vi "Script Flat to Rich Message Conversion.vi"(8 "error in (no error)":errorcluster, 9 "message metadata":T1, 10 "vi in":refnum<vi>, 11 "library in":refnum<vi>) -> (0 "error out":errorcluster, 2 "vi out":refnum<vi>, 3 "library out":refnum<vi>)   [LabVIEW 2019, in "gRPC Template Creation Utility.lvlib"]
uses:
  gRPC Template Creation Utility.lvlib
  TypeDefs/Message Metadata (Scripting).ctl
  TypeDefs/Message Element Metadata (Scripting).ctl
  TypeDefs/Message Element Type.ctl
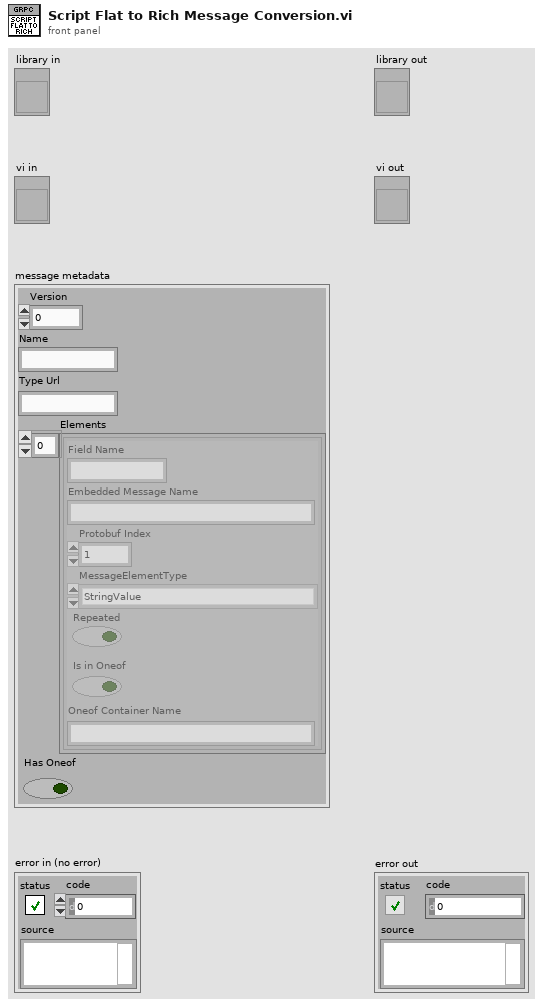
[diagram p1: front panel]
types:
  T1 = typedef "gRPC Template Creation Utility.lvlib/Message Metadata (Scripting).ctl" = cluster{"Version":i32, "Name":string, "Type Url":string, "Elements":T2[], "Has Oneof":bool}
  T2 = typedef "gRPC Template Creation Utility.lvlib/Message Element Metadata (Scripting).ctl" = cluster{"Field Name":string, "Embedded Message Name":string, "Protobuf Index":i32, "MessageElementType":T3, "Repeated":bool, "Is in Oneof":bool, "Oneof Container Name":string}
  T3 = typedef "gRPC Template Creation Utility.lvlib/Message Element Type.ctl" = enum32{"Int32Value", "FloatValue", "DoubleValue", "BoolValue", "StringValue", "MessageValue", "Int64Value", "UInt32Value", "UInt64Value", "EnumValue", "Bytes", "Fixed64", "Fixed32", "SFixed64", "SFixed32", "SInt64", "SInt32"}
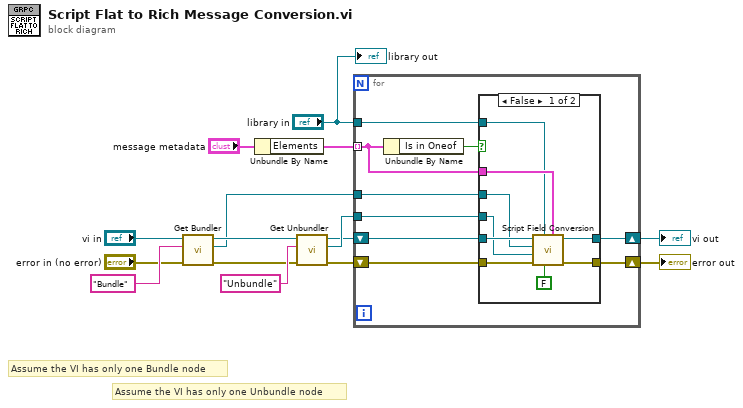
[diagram p0: block diagram]
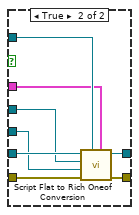
[diagram p2: hidden frame]
diagram:
  # "Assume the VI has only one Bundle node"
  # "Assume the VI has only one Unbundle node"
  n1 = call "Get Bundler.vi"("error in (no error)"="error in (no error)", "label"="Bundle" ("Class Name"), "owner vi in"="vi in") -> ("error out"=w7:errorcluster, "bundler ref"=w5:refnum<vi>, "owner vi out"=w8:refnum<vi>)  [unwired: 5 in, 1 out]
  n2 = Unbundle By Name("message metadata") -> ("Elements"=w3:T2[])
  n3 = call "Get Unbundler.vi"("error in (no error)"=w7, "Label"="Unbundle" ("Class Name"), "Owner VI in"=w8) -> ("error out"=w4:errorcluster, "Unbundler Refnum"=w10:refnum<vi>, "Owner VI out"=w9:refnum<vi>)  [unwired: 5 in, 1 out]
  n4 = for {
    tunnel: w3 -> [w16] mode=indexing
    tunnel: w5 -> [w24]
    tunnel: w10 -> [w23]
    shift-right: [w20] -> w15
    shift-left: w4 -> [w19]
    shift-right: [w18] -> w2
    shift-left: w9 -> [w22]
    tunnel: "library in" -> [w21]
    # "Iterate over the metadata elements (fields of a message) to wire the bundle and unbundle nodes"
    n5 = Unbundle By Name(w16) -> ("Is in Oneof"=w17:bool)
    n6 = case shown="False" w17 {
      tunnel: w19 -> [w33 w41]
      tunnel: [w31 w40] -> w20
      tunnel: w24 -> [w27 w37]
      tunnel: w23 -> [w26 w36]
      tunnel: w22 -> [w32 w38]
      tunnel: w21 -> [w28 w35]
      tunnel: [w30 w39] -> w18
      tunnel: w16 -> [w29 w34]
      frame False {
        # "Wire unbundle and bundle nodes whose terminals have the same name across serialization and message cluster."
        n7 = call "Script Field Conversion.vi"("element metadata"=w29, "rich to flat"=FALSE, "library in"=w28, "error in (no error)"=w33, "unbundler"=w26, "bundler"=w27, "vi in"=w32) -> ("error out"=w31:errorcluster, "vi out"=w30:refnum<vi>)  [unwired: 3 in]
      }
      frame True {
        # "Get the unbundle terminal whose name is <oneof container name>_selected_index.\nGet the bundle terminal whose name is <oneof container name> which is the class terminal."
        n8 = call "Script Flat to Rich Oneof Conversion.vi"("message element metadata"=w34, "library in"=w35, "error in (no error)"=w41, "unbundler"=w36, "bundler"=w37, "vi in"=w38) -> ("error out"=w40:errorcluster, "vi out"=w39:refnum<vi>)  [unwired: 4 in]
      }
    }
  }
  "error out" <- w15
  "vi out" <- w2
  "library out" <- "library in"
